vi "Pickball2.vi"   [LabVIEW 2016, in "Test.lvrbt"]
uses:
  Test.lvrbt
  <vilib>/NXT/Block Support/NXT_InputPort.ctl
  <vilib>/NXT/Subs/ColorSensorColors.ctl
  <vilib>/NXT/Hardware/Plugins/Tetrix DC Motor/TetrixDCMotorAddress.ctl
  <vilib>/NXT/Hardware/Plugins/Tetrix 180 deg Servo/Tetrix180ServoAddress.ctl
  <vilib>/NXT/NXTIO Xnodes/NXTIONodeSubVIs/TETRIX IO Move Servos.vi
  <vilib>/NXT/Dual Mode Library/Waits/Wait_Num.vi
  <vilib>/NXT/NXTIO Xnodes/NXTIONodeSubVIs/TETRIX IO Move DC Motors.vi
  <vilib>/NXT/NXTIO Xnodes/NXTIONodeSubVIs/TETRIX IO Stop DC Motors.vi
  <vilib>/NXT/Dual Mode Library/Waits/Wait_EV3_Ultrasonic_Centimeter_Closer.vi
  <vilib>/NXT/Dual Mode Library/Waits/Wait_EV3_Ultrasonic_Centimeters_Further.vi
  <vilib>/NXT/Dual Mode Library/Waits/Wait_EV3_Color_Color.vi
  <vilib>/NXT/NXTIO Xnodes/AddressXNode/NXTIOAddress.xnode
  <vilib>/NXT/Subs/LVHSConnector.ctl
  <vilib>/NXT/NXTIO Xnodes/NXTIOXNode/NXTIO.xnode
  <vilib>/NXT/LegoClasses/BrickReference/BrickReference.lvclass
types:
  T1 = typedef "NXT_InputPort.ctl" = u32
  T2 = typedef "ColorSensorColors.ctl" = enum16{"No Color", "Black", "Blue", "Green", "Yellow", "Red", "White", "Brown"}
  T3 = typedef "Tetrix180ServoAddress.ctl" = i32
  T4 = cluster{"Tetrix180Servo":T3, "Tetrix180Servo":T3, "Tetrix180Servo":T3, "Tetrix180Servo":T3, "Tetrix180Servo":T3}
  T5 = typedef "LVHSConnector.ctl" = refnum<class "BrickReference.lvclass">
  T6 = typedef "TetrixDCMotorAddress.ctl" = i32
diagram:
  w7 = T1 2 items=["Port 1", "Port 2", "Port 3", "Port 4"] ("Port (Port 1)")
  w90 = T1 1 items=["Port 1", "Port 2", "Port 3", "Port 4"] ("Port (Port 1)")
  w124 = T1 1 items=["Port 1", "Port 2", "Port 3", "Port 4"] ("Port (Port 1)")
  w131 = T1 1 items=["Port 1", "Port 2", "Port 3", "Port 4"] ("Port (Port 1)")
  w144 = T1 1 items=["Port 1", "Port 2", "Port 3", "Port 4"] ("Port (Port 1)")
  n1 = xnode "Motors"() -> ("Motor"=w102:T4)
  n2 = xnode "Move Servos"("Position 5"=u8 200, "Position 4"=u8 40, "Position 3"=u8 0, "Position 2"=u8 0, "Position 1"=u8 242, "Motors"=w102) -> ("NXT/EV3"=w95:T5)  [unwired: 1 in]
  n3 = xnode "Motors"() -> ("Motor"=w152:cluster{"TetrixDCMotor":T6, "TetrixDCMotor":T6})
  n4 = call-poly <vilib>:"PolyWait.vi"("Time (1 sec)"=sgl 1.0, "NXT/EV3"=w95) -> ("NXT/EV3"=w94:T5)  [unwired: 2 in]
  n5 = xnode "Move Motors"("Power/Speed 2"=i8 -100, "Power/Speed 1"=i8 -100, "Motors"=w152, "NXT/EV3"=w94) -> ("NXT/EV3"=w155:T5)
  n6 = call-poly <vilib>:"PolyWait.vi"("Time (1 sec)"=sgl 1.0, "NXT/EV3"=w155) -> ("NXT/EV3"=w153:T5)  [unwired: 2 in]
  n7 = xnode "Stop Motors"("Motors"=w152, "NXT/EV3"=w153) -> ("NXT/EV3"=w151:T5)
  n8 = xnode "Motors"() -> ("Motor"=w142:cluster{"TetrixDCMotor":T6, "TetrixDCMotor":T6})
  n9 = call-poly <vilib>:"PolyWait.vi"("Time (1 sec)"=sgl 1.0, "NXT/EV3"=w151) -> ("NXT/EV3"=w147:T5)  [unwired: 2 in]
  n10 = xnode "Move Motors"("Power/Speed 2"=i8 100, "Power/Speed 1"=i8 100, "Motors"=w142, "NXT/EV3"=w147) -> ("NXT/EV3"=w145:T5)
  n11 = call-poly <vilib>:"PolyWait.vi"("Centimeters (40)"=sgl 6.5 ("Time (1 sec)"), "NXT/EV3"=w145, "Port (Port 1)"=w144) -> ("NXT/EV3"=w143:T5)  [unwired: 1 in]
  n12 = xnode "Stop Motors"("Motors"=w142, "NXT/EV3"=w143) -> ("NXT/EV3"=w123:T5)
  n13 = xnode "Motors"() -> ("Motor"=w134:cluster{"TetrixDCMotor":T6, "TetrixDCMotor":T6})
  n14 = call-poly <vilib>:"PolyWait.vi"("Time (1 sec)"=sgl 1.0, "NXT/EV3"=w123) -> ("NXT/EV3"=w140:T5)  [unwired: 2 in]
  n15 = xnode "Move Motors"("Power/Speed 2"=i8 20, "Power/Speed 1"=i8 21, "Motors"=w134, "NXT/EV3"=w140) -> ("NXT/EV3"=w137:T5)
  n16 = call-poly <vilib>:"PolyWait.vi"("Centimeters (50)"=sgl 5.0, "NXT/EV3"=w137, "Port (Port 1)"=w131) -> ("NXT/EV3"=w135:T5)  [unwired: 1 in]
  n17 = xnode "Stop Motors"("Motors"=w134, "NXT/EV3"=w135) -> ("NXT/EV3"=w132:T5)
  n18 = xnode "Motors"() -> ("Motor"=w122:cluster{"TetrixDCMotor":T6, "TetrixDCMotor":T6})
  n19 = call-poly <vilib>:"PolyWait.vi"("Time (1 sec)"=sgl 1.0, "NXT/EV3"=w132) -> ("NXT/EV3"=w125:T5)  [unwired: 2 in]
  n20 = xnode "Move Motors"("Power/Speed 2"=i8 -5, "Power/Speed 1"=i8 -5, "Motors"=w122, "NXT/EV3"=w125) -> ("NXT/EV3"=w128:T5)
  n21 = call-poly <vilib>:"PolyWait.vi"("Centimeters (40)"=sgl 5.0, "NXT/EV3"=w128, "Port (Port 1)"=w124) -> ("NXT/EV3"=w127:T5)  [unwired: 1 in]
  n22 = xnode "Stop Motors"("Motors"=w122, "NXT/EV3"=w127) -> ("NXT/EV3"=w120:T5)
  n23 = xnode "Motors"() -> ("Motor"=w112:cluster{"TetrixDCMotor":T6, "TetrixDCMotor":T6})
  n24 = call-poly <vilib>:"PolyWait.vi"("Time (1 sec)"=sgl 1.0, "NXT/EV3"=w120) -> ("NXT/EV3"=w117:T5)  [unwired: 2 in]
  n25 = xnode "Move Motors"("Power/Speed 2"=i8 -5, "Power/Speed 1"=i8 -5, "Motors"=w112, "NXT/EV3"=w117) -> ("NXT/EV3"=w115:T5)
  n26 = xnode "Motors"() -> ("Sensor"=w114:T1)
  n27 = call-poly <vilib>:"PolyWait.vi"("Centimeters (40)"=sgl 18.5 ("Time (1 sec)"), "NXT/EV3"=w115, "Port (Port 1)"=w114) -> ("NXT/EV3"=w113:T5)  [unwired: 1 in]
  n28 = xnode "Stop Motors"("Motors"=w112, "NXT/EV3"=w113) -> ("NXT/EV3"=w110:T5)
  n29 = xnode "Motors"() -> ("Motor"=w103:cluster{"TetrixDCMotor":T6, "TetrixDCMotor":T6})
  n30 = call-poly <vilib>:"PolyWait.vi"("Time (1 sec)"=sgl 1.0, "NXT/EV3"=w110) -> ("NXT/EV3"=w109:T5)  [unwired: 2 in]
  n31 = xnode "Move Motors"("Power/Speed 2"=i8 -5, "Power/Speed 1"=i8 -5, "Motors"=w103, "NXT/EV3"=w109) -> ("NXT/EV3"=w105:T5)
  n32 = call-poly <vilib>:"PolyWait.vi"("Time (1 sec)"=sgl 0.6, "NXT/EV3"=w105) -> ("NXT/EV3"=w104:T5)  [unwired: 2 in]
  n33 = xnode "Stop Motors"("Motors"=w103, "NXT/EV3"=w104) -> ("NXT/EV3"=w1:T5)
  n34 = call-poly <vilib>:"PolyWait.vi"("Time (1 sec)"=sgl 1.0, "NXT/EV3"=w1) -> ("NXT/EV3"=w66:T5)  [unwired: 2 in]
  n35 = xnode "Motors"() -> ("Motor"=w85:T3)
  n36 = xnode "Move Servos"("Position 1"=u8 85, "Motors"=w85, "NXT/EV3"=w66) -> ("NXT/EV3"=w82:T5)
  n37 = call-poly <vilib>:"PolyWait.vi"("Time (1 sec)"=sgl 7.0, "NXT/EV3"=w82) -> ("NXT/EV3"=w79:T5)  [unwired: 2 in]
  n38 = xnode "Motors"() -> ("Motor"=w81:T3)
  n39 = xnode "Move Servos"("Position 1"=u8 227, "Motors"=w81, "NXT/EV3"=w79) -> ("NXT/EV3"=w77:T5)
  n40 = call-poly <vilib>:"PolyWait.vi"("Time (1 sec)"=sgl 0.5, "NXT/EV3"=w77) -> ("NXT/EV3"=w74:T5)  [unwired: 2 in]
  n41 = xnode "Motors"() -> ("Motor"=w76:T3)
  n42 = xnode "Move Servos"("Position 1"=u8 20, "Motors"=w76, "NXT/EV3"=w74) -> ("NXT/EV3"=w72:T5)
  n43 = call-poly <vilib>:"PolyWait.vi"("Time (1 sec)"=sgl 1.5, "NXT/EV3"=w72) -> ("NXT/EV3"=w69:T5)  [unwired: 2 in]
  n44 = xnode "Motors"() -> ("Motor"=w70:T3)
  n45 = xnode "Move Servos"("Position 1"=u8 98, "Motors"=w70, "NXT/EV3"=w69) -> ("NXT/EV3"=w68:T5)
  n46 = xnode "Motors"() -> ("Motor"=w88:cluster{"TetrixDCMotor":T6, "TetrixDCMotor":T6})
  n47 = call-poly <vilib>:"PolyWait.vi"("Time (1 sec)"=sgl 1.0, "NXT/EV3"=w68) -> ("NXT/EV3"=w86:T5)  [unwired: 2 in]
  n48 = xnode "Move Motors"("Power/Speed 2"=i8 5, "Power/Speed 1"=i8 5, "Motors"=w88, "NXT/EV3"=w86) -> ("NXT/EV3"=w91:T5)
  n49 = call-poly <vilib>:"PolyWait.vi"("Centimeters (50)"=sgl 5.0, "NXT/EV3"=w91, "Port (Port 1)"=w90) -> ("NXT/EV3"=w89:T5)  [unwired: 1 in]
  n50 = xnode "Stop Motors"("Motors"=w88, "NXT/EV3"=w89) -> ("NXT/EV3"=w63:T5)
  n51 = call-poly <vilib>:"PolyWait.vi"("Time (1 sec)"=sgl 1.0, "NXT/EV3"=w63) -> ("NXT/EV3"=w60:T5)  [unwired: 2 in]
  n52 = xnode "Motors"() -> ("Motor"=w61:T3)
  n53 = xnode "Move Servos"("Position 1"=u8 67, "Motors"=w61, "NXT/EV3"=w60) -> ("NXT/EV3"=w58:T5)
  n54 = call-poly <vilib>:"PolyWait.vi"("Time (1 sec)"=sgl 1.0, "NXT/EV3"=w58) -> ("NXT/EV3"=w55:T5)  [unwired: 2 in]
  n55 = xnode "Motors"() -> ("Motor"=w56:T3)
  n56 = xnode "Move Servos"("Position 1"=u8 240, "Motors"=w56, "NXT/EV3"=w55) -> ("NXT/EV3"=w53:T5)
  n57 = xnode "Motors"() -> ("Motor"=w46:cluster{"TetrixDCMotor":T6, "TetrixDCMotor":T6})
  n58 = call-poly <vilib>:"PolyWait.vi"("Time (1 sec)"=sgl 1.0, "NXT/EV3"=w53) -> ("NXT/EV3"=w52:T5)  [unwired: 2 in]
  n59 = xnode "Move Motors"("Power/Speed 2"=i8 -100, "Power/Speed 1"=i8 -100, "Motors"=w46, "NXT/EV3"=w52) -> ("NXT/EV3"=w48:T5)
  n60 = call-poly <vilib>:"PolyWait.vi"("Time (1 sec)"=sgl 1.0, "NXT/EV3"=w48) -> ("NXT/EV3"=w47:T5)  [unwired: 2 in]
  n61 = xnode "Stop Motors"("Motors"=w46, "NXT/EV3"=w47) -> ("NXT/EV3"=w44:T5)
  n62 = xnode "Motors"() -> ("Motor"=w37:cluster{"TetrixDCMotor":T6, "TetrixDCMotor":T6})
  n63 = call-poly <vilib>:"PolyWait.vi"("Time (1 sec)"=sgl 1.0, "NXT/EV3"=w44) -> ("NXT/EV3"=w41:T5)  [unwired: 2 in]
  n64 = xnode "Move Motors"("Power/Speed 2"=i8 -100, "Power/Speed 1"=i8 -100, "Motors"=w37, "NXT/EV3"=w41) -> ("NXT/EV3"=w39:T5)
  n65 = call-poly <vilib>:"PolyWait.vi"("Time (1 sec)"=sgl 1.0, "NXT/EV3"=w39) -> ("NXT/EV3"=w38:T5)  [unwired: 2 in]
  n66 = xnode "Stop Motors"("Motors"=w37, "NXT/EV3"=w38) -> ("NXT/EV3"=w35:T5)
  n67 = call-poly <vilib>:"PolyWait.vi"("Time (1 sec)"=sgl 1.0, "NXT/EV3"=w35) -> ("NXT/EV3"=w32:T5)  [unwired: 2 in]
  n68 = xnode "Motors"() -> ("Motor"=w33:T3)
  n69 = xnode "Move Servos"("Position 1"=u8 0, "Motors"=w33, "NXT/EV3"=w32) -> ("NXT/EV3"=w30:T5)
  n70 = call-poly <vilib>:"PolyWait.vi"("Time (1 sec)"=sgl 1.0, "NXT/EV3"=w30) -> ("NXT/EV3"=w27:T5)  [unwired: 2 in]
  n71 = xnode "Motors"() -> ("Motor"=w28:T3)
  n72 = xnode "Move Servos"("Position 1"=u8 242, "Motors"=w28, "NXT/EV3"=w27) -> ("NXT/EV3"=w25:T5)
  n73 = call-poly <vilib>:"PolyWait.vi"("Time (1 sec)"=sgl 1.0, "NXT/EV3"=w25) -> ("NXT/EV3"=w22:T5)  [unwired: 2 in]
  n74 = xnode "Motors"() -> ("Motor"=w23:T3)
  n75 = xnode "Move Servos"("Position 1"=u8 0, "Motors"=w23, "NXT/EV3"=w22) -> ("NXT/EV3"=w13:T5)
  n76 = xnode "Motors"() -> ("Motor"=w5:cluster{"TetrixDCMotor":T6, "TetrixDCMotor":T6})
  n77 = call-poly <vilib>:"PolyWait.vi"("Time (1 sec)"=sgl 1.5, "NXT/EV3"=w13) -> ("NXT/EV3"=w12:T5)  [unwired: 2 in]
  n78 = xnode "Move Motors"("Power/Speed 2"=i8 10, "Power/Speed 1"=i8 10, "Motors"=w5, "NXT/EV3"=w12) -> ("NXT/EV3"=w9:T5)
  n79 = call-poly <vilib>:"PolyWait.vi"("Color (Red)"=ColorSensorColors."Black", "NXT/EV3"=w9, "Port (Port 1)"=w7) -> ("NXT/EV3"=w6:T5)  [unwired: 1 in]
  n80 = xnode "Stop Motors"("Motors"=w5, "NXT/EV3"=w6) -> ("NXT/EV3"=w3:T5)
  n81 = call-poly <vilib>:"PolyWait.vi"("Time (1 sec)"=sgl 1.5, "NXT/EV3"=w3) -> ("NXT/EV3"=w2:T5)  [unwired: 2 in]
  n82 = xnode "Motors"() -> ("Motor"=w20:T3)
  n83 = xnode "Move Servos"("Position 1"=u8 118, "Motors"=w20, "NXT/EV3"=w2) -> ("NXT/EV3"=w18:T5)
  n84 = call-poly <vilib>:"PolyWait.vi"("Time (1 sec)"=sgl 2.0, "NXT/EV3"=w18) -> ("NXT/EV3"=w15:T5)  [unwired: 2 in]
  n85 = xnode "Motors"() -> ("Motor"=w16:T3)
  n86 = xnode "Move Servos"("Position 1"=u8 40, "Motors"=w16, "NXT/EV3"=w15) -> ()  [unwired: 1 out]
